vi "Reference_select.vi"(4 "Ref_Sel(Int/Ext)":enum16{"Int", "Ext"}(ring), 6 "INT_Ref_Sel":enum16{"Int_Ref_1P65", "Int_Ref_2P5"}(ring)=enum."Int_Ref_2P5", 8 "error in":errorcluster, 10 "Core Number":u16=1 min=1 step=1, 11 "Port Number":u16=1444) -> (0 "error out":errorcluster)   [LabVIEW 2019]
uses:
  <userlib>/_TI-LA/Reusable/CCS/APIs/Data/Polymorphics/Write Data To Symbol - U16.vi
  <userlib>/_TI-LA/Reusable/CCS/APIs/CCS.lvlib
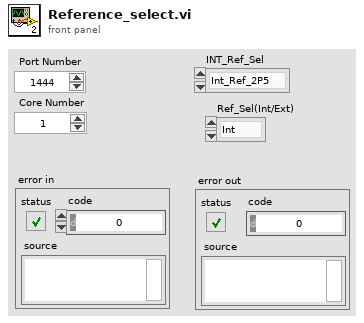
[diagram p1: front panel]
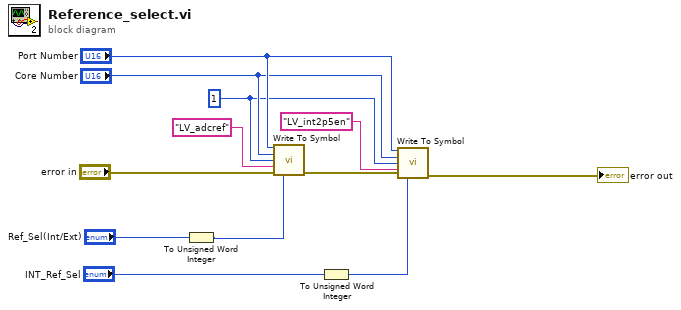
[diagram p0: block diagram]
diagram:
  w6 = 1 ("Page")
  n1 = To Unsigned Word Integer(number="Ref_Sel(Int/Ext)") -> (unsigned 16bit integer=w2:u16)
  n2 = call-poly <userlib>:"Write To Symbol.vi"("Port Number"="Port Number", "Core Number"="Core Number", "Page"=w6, "Symbol Name"="LV_adcref", "error in"="error in", "Write Data"=w2) -> ("error out"=w12:errorcluster)  [unwired: 7 in, 2 out]
  n3 = To Unsigned Word Integer(number="INT_Ref_Sel") -> (unsigned 16bit integer=w3:u16)
  n4 = call-poly <userlib>:"Write To Symbol.vi"("Port Number"="Port Number", "Core Number"="Core Number", "Page"=w6, "Symbol Name"="LV_int2p5en", "error in"=w12, "Write Data"=w3) -> ("error out"=→"error out":errorcluster)  [unwired: 7 in, 2 out]
